vi "RP Demo Client.vi"(8 "Error In":errorcluster, 11 "VISA resource name":refnum<visa-resource-name>="RP100") -> (0 "Error Out":errorcluster)   [LabVIEW 2016]
panel:
  out "FPGA bitfile tag":u16
  out "IDN response":u32=1 format="0x%x (%d)"
  in  "bytes to read":i32=4
  in  "Command":u64=1
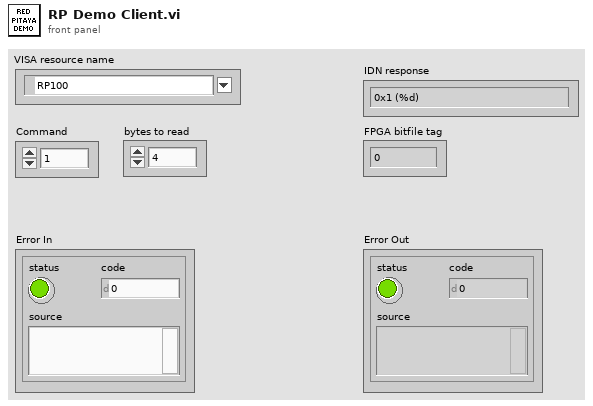
[diagram p1: front panel]
types:
  T1 = enum16{"big-endian, network order", "native, host order", "little-endian"}
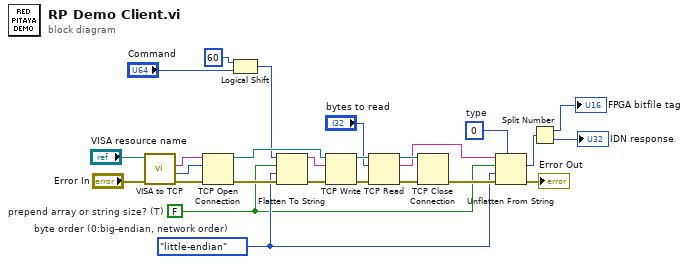
[diagram p0: block diagram]
diagram:
  w9 = u32 0  # type
  w10 = T1."little-endian"  # byte order (0:big-endian, network order)
  w1 = FALSE  # prepend array or string size? (T)
  n1 = call "VISA to TCP.vi"("Error In"="Error In", "VISA resource name"="VISA resource name") -> ("Error Out"=w24:errorcluster, "Port"=w22:u16, "Hostname"=w23:string)  [unwired: 6 in, 1 out]
  n2 = TCP Open Connection(address=w23, remote port or service name=w22, error in (no error)=w24) -> (connection ID=w19:refnum<k5>, error out=w21:errorcluster)  [unwired: 2 in]
  n3 = Logical Shift(y=i16 60, x="Command") -> (x << y=w4:u64)
  n4 = Flatten To String(anything=w4, prepend array or string size? (T)=w1, byte order (0:big-endian, network order)=w10, error in (no error)=w21) -> (data string=w18:string, error out=w20:errorcluster)  [unwired: 1 out]
  n5 = TCP Write(connection ID=w19, data in=w18, error in (no error)=w20) -> (connection ID out=w16:refnum<k5>, error out=w17:errorcluster)  [unwired: 1 in, 1 out]
  n6 = TCP Read(connection ID=w16, bytes to read="bytes to read", error in (no error)=w17) -> (connection ID out=w13:refnum<k5>, data out=w12:string, error out=w14:errorcluster)  [unwired: 2 in]
  n7 = TCP Close Connection(connection ID=w13, error in (no error)=w14) -> (error out=w11:errorcluster)  [unwired: 1 in, 1 out]
  n8 = Unflatten From String(type=w9, binary string=w12, data includes array or string size? (T)=w1, byte order (0:big-endian, network order)=w10, error in (no error)=w11) -> (value=w8:u32, error out=→"Error Out":errorcluster)  [unwired: 1 out]
  n9 = Split Number(x=w8) -> (hi(x)=→"FPGA bitfile tag":u16, lo(x)=→"IDN response":u16)
